vi "Add Images to Report.vi"(8 "error in (no error)":errorcluster, 10 "Folder (temp directory)":path, 11 "Control References":refnum<vi>[](array[refnum])) -> (0 "error out":errorcluster, 3 "Report String":string)   [LabVIEW 2011]
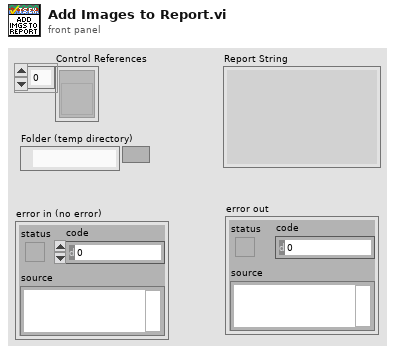
[diagram p1: front panel]
types:
  T1 = typedef "imagedata.ctl" = cluster{"image type":i32, "image depth":i32, "image":u8[], "mask":u8[], "colors":u32[], "Rectangle":cluster{"left":i16, "top":i16, "right":i16, "bottom":i16}}
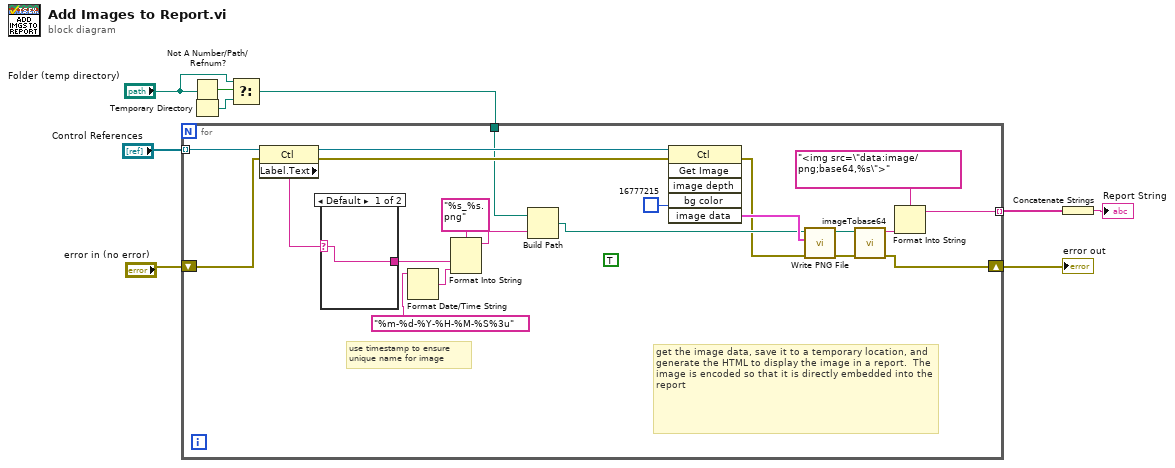
[diagram p0: block diagram]
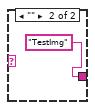
[diagram p2: hidden frame]
diagram:
  n1 = Not A Number/Path/Refnum?(number/path/refnum="Folder (temp directory)") -> (NaN/Path/Refnum?=w4:bool)
  n2 = Temporary Directory() -> (w2:path)
  n3 = Select(t="Folder (temp directory)", s=w4, f=w2) -> (s? t:f=w3:path)
  n4 = for {
    tunnel: "Control References" -> [w25] mode=indexing
    tunnel: [w27] -> w8 mode=indexing
    shift-right: [w10] -> w5
    shift-left: "error in (no error)" -> [w23]
    tunnel: w3 -> [w14]
    (unwired) TRUE ("Always Overwrite")
    # "get the image data, save it to a temporary location, and generate the HTML to display the image in a report.  The image is encoded so that it is directly embedded into the report"
    # "use timestamp to ensure \nunique name for image"
    n5 = property class="Ctl"(reference=w25, error in=w23) -> (reference out=w21:refnum<vi>, error out=w22:errorcluster, "Label.Text"=w18:string)
    n6 = case shown="Default" w18 {
      selector: w18 -> [w31 _]
      tunnel: [w31 "TestImg"] -> w17
      frame Default {
      }
      frame "" {
      }
    }
    n7 = Format Date/Time String(time format string (%c)="%m-%d-%Y-%H-%M-%S%3u") -> (date/time string=w16:string)  [unwired: 2 in]
    n8 = Format Into String(format string="%s_%s.png", w17, w16) -> (resulting string=w19:string)  [unwired: 2 in, 1 out]
    n9 = Build Path(base path=w14, name or relative path=w19) -> (appended path=w29:path)
    n10 = invoke class="Ctl" method="Get Image"(reference=w21, error in=w22, "bg color"=u32 16777215) -> (error out=w20:errorcluster, "image data"=w30:T1)  [unwired: 3 in, 4 out]
    n11 = call <vilib>:"Write PNG File.vi"("error in (no error)"=w20, "image data"=w30, "path to PNG file"=w29) -> ("error out"=w11:errorcluster, "path"=w13:path)  [unwired: 7 in]
    n12 = call "imageTobase64.vi"("error in (no error)"=w11, "path to PNG file"=w13) -> ("error out"=w10:errorcluster, "string out (base64-encoded)"=w12:string)  [unwired: 8 in]
    n13 = Format Into String(format string="<img src=\"data:image/png;base64,%s\">", w12) -> (resulting string=w27:string)  [unwired: 2 in, 1 out]
  }
  "error out" <- w5
  n14 = Concatenate Strings(w8) -> (→"Report String":string)
